vi "Create Serial Input Channel CSI-2 IO x2.vi"() -> (4 "serial input csi-2 io x2":T4)   [LabVIEW 2020, in "GettingStarted_Acq_Tap_148X_FPGA.lvlib"]
uses:
  GettingStarted_Acq_Tap_148X_FPGA.lvlib
  Types/Serial Input Channel IO.ctl
  Types/Serial Input Channel IO 32b.ctl
  Types/Serial Input Channel IO 64b.ctl
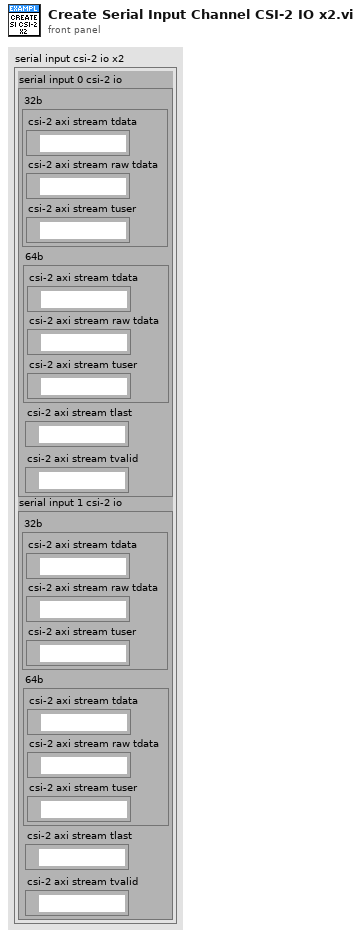
[diagram p1: front panel]
types:
  T1 = typedef "GettingStarted_Acq_Tap_148X_FPGA.lvlib/Serial Input Channel IO.ctl" = cluster{"32b":T2, "64b":T3, "csi-2 axi stream tlast":refnum<k21>, "csi-2 axi stream tvalid":refnum<k21>}
  T2 = typedef "GettingStarted_Acq_Tap_148X_FPGA.lvlib/Serial Input Channel IO 32b.ctl" = cluster{"csi-2 axi stream tdata":refnum<k21>, "csi-2 axi stream raw tdata":refnum<k21>, "csi-2 axi stream tuser":refnum<k21>}
  T3 = typedef "GettingStarted_Acq_Tap_148X_FPGA.lvlib/Serial Input Channel IO 64b.ctl" = cluster{"csi-2 axi stream tdata":refnum<k21>, "csi-2 axi stream raw tdata":refnum<k21>, "csi-2 axi stream tuser":refnum<k21>}
  T4 = cluster{"serial input 0 csi-2 io":T1, "serial input 1 csi-2 io":T1}
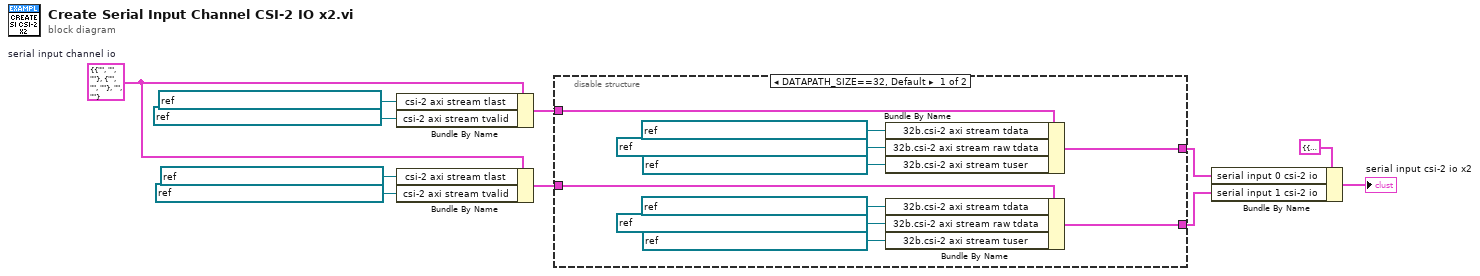
[diagram p0: block diagram]
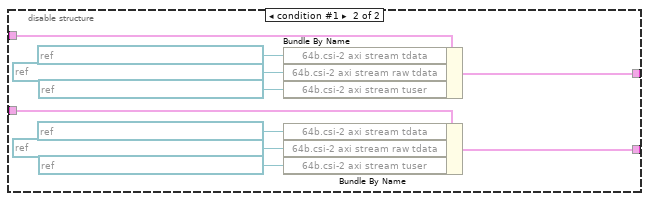
[diagram p2: hidden frame]
diagram:
  w9 = T1 {"32b"={"csi-2 axi stream tdata"="", "csi-2 axi stream raw tdata"="", "csi-2 axi stream tuser"=""}, "64b"={"csi-2 axi stream tdata"="", "csi-2 axi stream raw tdata"="", "csi-2 axi stream tuser"=""}, "csi-2 axi stream tlast"="", "csi-2 axi stream tvalid"=""}  # serial input channel io
  n1 = Bundle By Name(cluster=w9, "csi-2 axi stream tlast"=refnum<k21> "IO Socket\\SI 0 CSI-2 AXI Stream TLast" ("FPGA I/O In"), "csi-2 axi stream tvalid"=refnum<k21> "IO Socket\\SI 0 CSI-2 AXI Stream TValid" ("FPGA I/O In")) -> (w4:T1)
  n2 = Bundle By Name(cluster=w9, "csi-2 axi stream tlast"=refnum<k21> "IO Socket\\SI 1 CSI-2 AXI Stream TLast" ("FPGA I/O In"), "csi-2 axi stream tvalid"=refnum<k21> "IO Socket\\SI 1 CSI-2 AXI Stream TValid" ("FPGA I/O In")) -> (w3:T1)
  n3 = disable-structure shown="DATAPATH_SIZE==32, Default" {
    disable-tunnel: w4 -> [w21 w29]
    disable-tunnel: w3 -> [w20 w24]
    disable-tunnel: [w13 w23] -> w2
    disable-tunnel: [w12 w22] -> w1
    frame condition #0 (active) {
      n4 = Bundle By Name(cluster=w21, "32b.csi-2 axi stream tdata"=refnum<k21> "IO Socket\\SI 0 CSI-2 AXI Stream TData" ("FPGA I/O In"), "32b.csi-2 axi stream raw tdata"=refnum<k21> "IO Socket\\SI 0 CSI-2 AXI Stream Raw TData" ("FPGA I/O In"), "32b.csi-2 axi stream tuser"=refnum<k21> "IO Socket\\SI 0 CSI-2 AXI Stream TUser" ("FPGA I/O In")) -> (w13:T1)
      n5 = Bundle By Name(cluster=w20, "32b.csi-2 axi stream tdata"=refnum<k21> "IO Socket\\SI 1 CSI-2 AXI Stream TData" ("FPGA I/O In"), "32b.csi-2 axi stream raw tdata"=refnum<k21> "IO Socket\\SI 1 CSI-2 AXI Stream Raw TData" ("FPGA I/O In"), "32b.csi-2 axi stream tuser"=refnum<k21> "IO Socket\\SI 1 CSI-2 AXI Stream TUser" ("FPGA I/O In")) -> (w12:T1)
    }
    frame condition #1 {
      n6 = Bundle By Name(cluster=w29, "64b.csi-2 axi stream tdata"=refnum<k21> "IO Socket\\SI 0 CSI-2 AXI Stream TData" ("FPGA I/O In"), "64b.csi-2 axi stream raw tdata"=refnum<k21> "IO Socket\\SI 0 CSI-2 AXI Stream Raw TData" ("FPGA I/O In"), "64b.csi-2 axi stream tuser"=refnum<k21> "IO Socket\\SI 0 CSI-2 AXI Stream TUser" ("FPGA I/O In")) -> (w23:T1)
      n7 = Bundle By Name(cluster=w24, "64b.csi-2 axi stream tdata"=refnum<k21> "IO Socket\\SI 1 CSI-2 AXI Stream TData" ("FPGA I/O In"), "64b.csi-2 axi stream raw tdata"=refnum<k21> "IO Socket\\SI 1 CSI-2 AXI Stream Raw TData" ("FPGA I/O In"), "64b.csi-2 axi stream tuser"=refnum<k21> "IO Socket\\SI 1 CSI-2 AXI Stream TUser" ("FPGA I/O In")) -> (w22:T1)
    }
  }
  n8 = Bundle By Name(cluster=T4 {"serial input 0 csi-2 io"={"32b"={"csi-2 axi stream tdata"="", "csi-2 axi stream raw tdata"="", "csi-2 axi stream tuser"=""}, "64b"={"csi-2 axi stream tdata"="", "csi-2 axi stream raw tdata"="", "csi-2 axi stream tuser"=""}, "csi-2 axi stream tlast"="", "csi-2 axi stream tvalid"=""}, "serial input 1 csi-2 io"={"32b"={"csi-2 axi stream tdata"="", "csi-2 axi stream raw tdata"="", "csi-2 axi stream tuser"=""}, "64b"={"csi-2 axi stream tdata"="", "csi-2 axi stream raw tdata"="", "csi-2 axi stream tuser"=""}, "csi-2 axi stream tlast"="", "csi-2 axi stream tvalid"=""}} ("serial input csi-2 io x2"), "serial input 0 csi-2 io"=w2, "serial input 1 csi-2 io"=w1) -> (→"serial input csi-2 io x2":T4)
